vi "Post-Install Library Setup.vi"(10 "Variant":variant) -> (0 "error out":errorcluster)   [LabVIEW 2014]
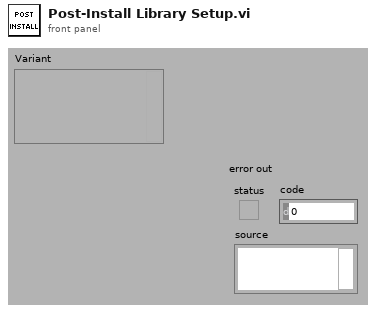
[diagram p1: front panel]
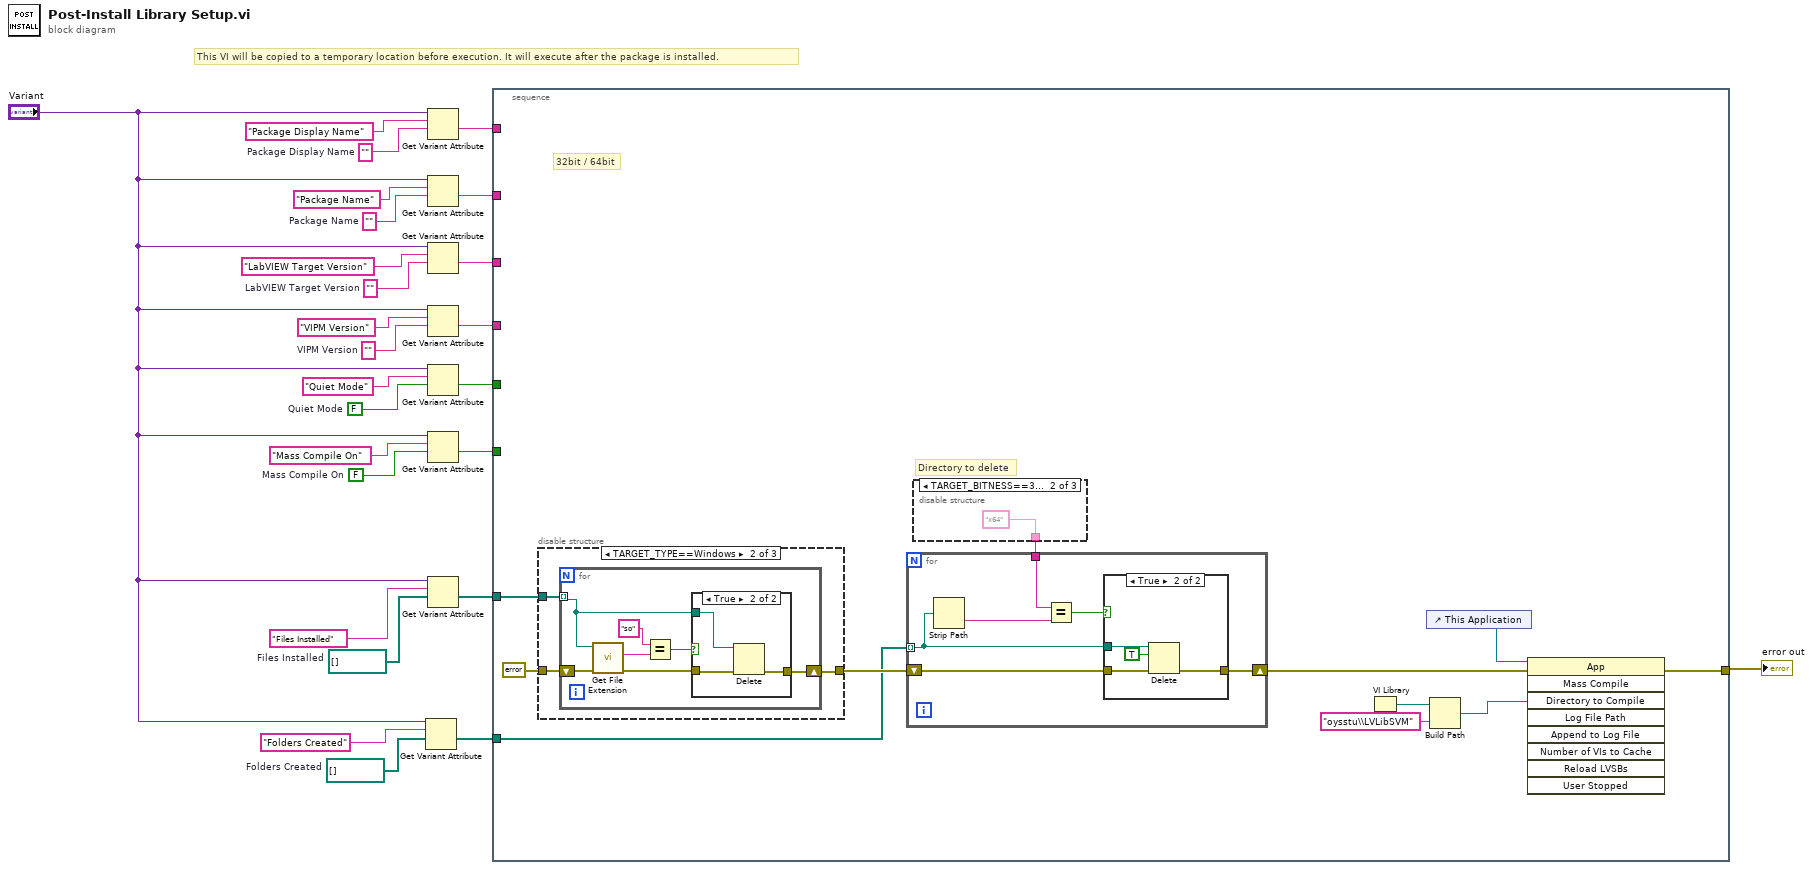
[diagram p0: block diagram]
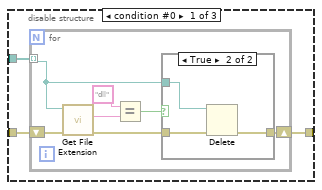
[diagram p3: hidden frame]
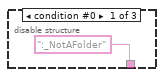
[diagram p7: hidden frame]
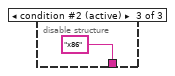
[diagram p8: hidden frame]
diagram:
  w2 = path[] []  # Folders Created
  w3 = path[] []  # Files Installed
  w9 = FALSE  # Mass Compile On
  w10 = ""  # Package Display Name
  w17 = FALSE  # Quiet Mode
  w20 = ""  # VIPM Version
  w22 = ""  # LabVIEW Target Version
  w24 = ""  # Package Name
  # "This VI will be copied to a temporary location before execution. It will execute after the package is installed."
  n1 = Get Variant Attribute(Variant="Variant", name="Folders Created", default value (empty Variant)=w2) -> (value=w7:path[])  [unwired: 1 in, 3 out]
  n2 = Get Variant Attribute(Variant="Variant", name="Package Display Name", default value (empty Variant)=w10) -> (value=w16:string)  [unwired: 1 in, 3 out]
  n3 = Get Variant Attribute(Variant="Variant", name="Package Name", default value (empty Variant)=w24) -> (value=w15:string)  [unwired: 1 in, 3 out]
  n4 = Get Variant Attribute(Variant="Variant", name="LabVIEW Target Version", default value (empty Variant)=w22) -> (value=w14:string)  [unwired: 1 in, 3 out]
  n5 = Get Variant Attribute(Variant="Variant", name="VIPM Version", default value (empty Variant)=w20) -> (value=w13:string)  [unwired: 1 in, 3 out]
  n6 = Get Variant Attribute(Variant="Variant", name="Quiet Mode", default value (empty Variant)=w17) -> (value=w12:bool)  [unwired: 1 in, 3 out]
  n7 = Get Variant Attribute(Variant="Variant", name="Mass Compile On", default value (empty Variant)=w9) -> (value=w11:bool)  [unwired: 1 in, 3 out]
  n8 = Get Variant Attribute(Variant="Variant", name="Files Installed", default value (empty Variant)=w3) -> (value=w6:path[])  [unwired: 1 in, 3 out]
  n9 = stacked-sequence {
    tunnel: w16 -> [_]
    tunnel: w15 -> [_]
    tunnel: w14 -> [_]
    tunnel: w13 -> [_]
    tunnel: w12 -> [_]
    tunnel: w11 -> [_]
    tunnel: w6 -> [w36]
    tunnel: w7 -> [w30]
    tunnel: [w32] -> w1
    frame #0 {
      # "Directory to delete"
      # "32bit / 64bit"
      n10 = disable-structure shown="TARGET_TYPE==Windows" {
        disable-tunnel: errorcluster {"status"=FALSE, "code"=0, "source"=""} ("error out") -> [w51 w65 w77]
        disable-tunnel: w36 -> [w50 w64 _]
        disable-tunnel: [w49 w63 w77] -> w35
        frame condition #0 {
          n11 = for {
            tunnel: w50 -> [w52] mode=indexing
            shift-right: [w53] -> w49
            shift-left: w51 -> [w58]
            n12 = call <vilib>:"Get File Extension.vi"("error in (no error)"=w58, "file"=w52) -> ("error out"=w57:errorcluster, "lowercase file extension"=w56:string)  [unwired: 6 in, 2 out]
            n13 = Equal?(x="dll", y=w56) -> (x = y?=w55:bool)
            n14 = case shown="True" w55 {
              tunnel: w57 -> [w59 w62]
              tunnel: [w59 w61] -> w53
              tunnel: w52 -> [_ w60]
              frame False {
              }
              frame True {
                n15 = Delete(path (use dialog)=w60, error in=w62) -> (error out=w61:errorcluster)  [unwired: 3 in, 2 out]
              }
            }
          }
        }
        frame condition #1 (active) {
          n16 = for {
            tunnel: w64 -> [w66] mode=indexing
            shift-right: [w67] -> w63
            shift-left: w65 -> [w72]
            n17 = call <vilib>:"Get File Extension.vi"("error in (no error)"=w72, "file"=w66) -> ("error out"=w71:errorcluster, "lowercase file extension"=w70:string)  [unwired: 6 in, 2 out]
            n18 = Equal?(x="so", y=w70) -> (x = y?=w69:bool)
            n19 = case shown="True" w69 {
              tunnel: w71 -> [w73 w76]
              tunnel: [w73 w75] -> w67
              tunnel: w66 -> [_ w74]
              frame False {
              }
              frame True {
                n20 = Delete(path (use dialog)=w74, error in=w76) -> (error out=w75:errorcluster)  [unwired: 3 in, 2 out]
              }
            }
          }
        }
        frame condition #2 {
        }
      }
      n21 = disable-structure shown="TARGET_BITNESS==32" {
        disable-tunnel: [":_NotAFolder" "x64" "x86"] -> w34
        frame condition #0 {
        }
        frame condition #1 {
        }
        frame condition #2 (active) {
        }
      }
      n22 = for {
        tunnel: w30 -> [w39] mode=indexing
        tunnel: w34 -> [w43]
        shift-right: [w38] -> w31
        shift-left: w35 -> [w41]
        n23 = Strip Path(path=w39) -> (name=w42:string)  [unwired: 1 out]
        n24 = Equal?(x=w43, y=w42) -> (x = y?=w40:bool)
        n25 = case shown="True" w40 {
          tunnel: w41 -> [w44 w48]
          tunnel: w39 -> [_ w47]
          tunnel: [w44 w46] -> w38
          frame False {
          }
          frame True {
            n26 = Delete(path (use dialog)=w47, entire hierarchy (F)=TRUE, error in=w48) -> (error out=w46:errorcluster)  [unwired: 2 in, 2 out]
          }
        }
      }
      n27 = VI Library() -> (path=w29:path)
      n28 = control-ref of="This Application"() -> (w33:refnum<vi>)
      n29 = Build Path(base path=w29, name or relative path="oysstu\\LVLibSVM") -> (appended path=w27:path)
      n30 = invoke class="App" method="Mass Compile"(reference=w33, error in=w31, "Directory to Compile"=w27) -> (error out=w32:errorcluster)  [unwired: 6 in, 8 out]
    }
  }
  "error out" <- w1
